vi "VMS_CameraRotator_Responder.vi"() -> ()   [LabVIEW 2018]
uses:
  <vilib>/rvi/Emulation/niFpgaGetClockAttributes.vi
  <vilib>/rvi/Emulation/niFpgaSctlEmulationGetInTimedLoop.vi
  <vilib>/rvi/Emulation/niFpgaEmulationReportErrorSimple.vi
  <vilib>/rvi/eio/common/nirviEmuTemplateMethod_errors.vi
  <vilib>/rvi/interface/RandomDataEmulation/niFpgaRandomDataHandleErrors.vi
  <vilib>/rvi/Emulation/niFpgaProcessEmulError.vi
  <vilib>/rvi/Emulation/niFpgaCriticalErrorInLSC.vi
  <vilib>/rvi/occurrence/nirviWaitOnOccurrenceBase.vi
  <vilib>/eio/EIOMethodNode/EIOMethodNode.xnode
  <vilib>/rvi/DataTransferAndStorage/Container/XNode/niFpgaContainer.xnode
  <vilib>/rvi/interface/RandomDataEmulation/nirviRandomDataFpgaReadWriteTemplate.vi
  <vilib>/eio/EIONode/EIONode.xnode
panel:
  out "Chassis Temperature":fxp<+/-,32,16>
  out "FIFO full":bool
  in  "Output type":i16
  in  "Period (ms)":u32=5
  out "Ready":bool
  out "Ticks":u64
  out "Timeouted":bool
  out "Stopped":bool
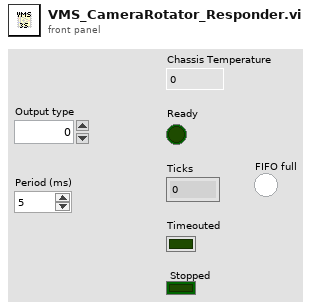
[diagram p1: front panel]
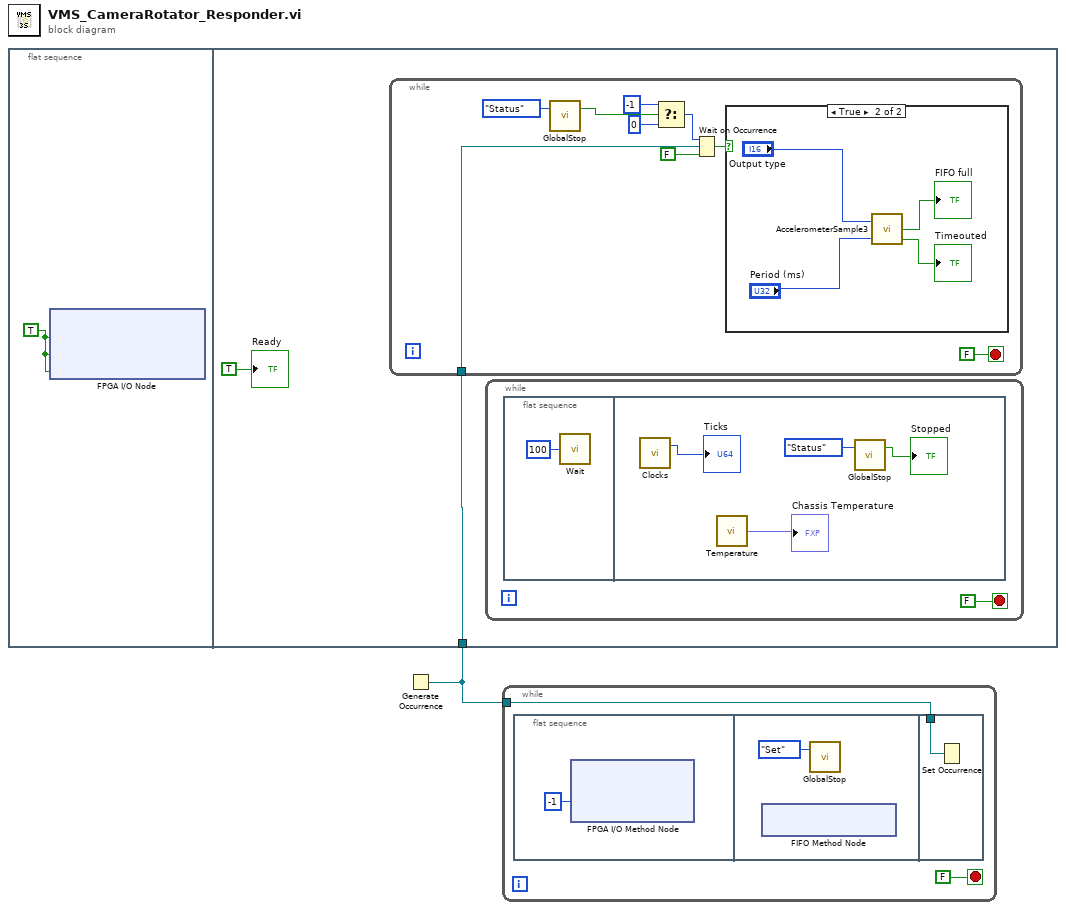
[diagram p0: block diagram]
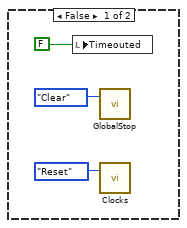
[diagram p2: hidden frame]
diagram:
  n1 = flat-sequence {
    tunnel: w1 -> [w3]
    frame #0 {
      w2 = TRUE ("Accelerometer5/Start")
      n2 = xnode "FPGA I/O Node"("Accelerometer1/Start"=w2, "Accelerometer2/Start"=w2, "Accelerometer3/Start"=w2) -> ()  [unwired: 3 in, 3 out]
    }
    frame #1 {
      n3 = while {
        tunnel: w3 -> [w17]
        stop <- FALSE stop-if-true
        n4 = call "GlobalStop.vi"("Enum"=enum16{"Clear", "Set", "Status"}."Status") -> ("Boolean"=w11:bool)  [unwired: 1 in, 1 out]
        n5 = Select(t=-1, s=w11, f=0) -> (s? t:f=w15:i32)
        n6 = Wait on Occurrence(1:FALSE ("ignore previous (T)"), 2:w17, 3:w15) -> (0:w18:bool)
        n7 = case shown="True" w18 {
          frame False {
            n8 = local write "Timeouted"(FALSE ("Timeouted")) -> ()
            n9 = call "GlobalStop.vi"("Enum"=enum16{"Clear", "Set", "Status"}."Clear") -> ()  [unwired: 1 in, 2 out]
            n10 = call "Clocks.vi"("Enum"=enum16{"Reset", "Increment", "Get"}."Reset") -> ()  [unwired: 1 in, 2 out]
          }
          frame True {
            n11 = call "AccelerometerSample3.vi"("Output type"="Output type", "Period (ms)"="Period (ms)") -> ("FIFO full"=→"FIFO full":bool, "Timeouted"=→"Timeouted":bool)  [unwired: 1 out]
          }
        }
      }
      n12 = while {
        stop <- FALSE stop-if-true
        n13 = flat-sequence {
          frame #0 {
            n14 = call "Wait"("Count(mSec)"=u32 100) -> ()  [unwired: 1 out]
          }
          frame #1 {
            n15 = call "Clocks.vi"() -> ("Clock"=→"Ticks":u64)  [unwired: 2 in, 1 out]
            n16 = call "Temperature.vi"() -> ("Mean temperature"=→"Chassis Temperature":fxp<+/-,32,16>)  [unwired: 1 in]
            n17 = call "GlobalStop.vi"("Enum"=enum16{"Clear", "Set", "Status"}."Status") -> ("Boolean"=→"Stopped":bool)  [unwired: 1 in, 1 out]
          }
        }
      }
      "Ready" <- TRUE ("Ready")
    }
  }
  n18 = Generate Occurrence() -> (w1:refnum<k4>)
  n19 = while {
    tunnel: w1 -> [w27]
    stop <- FALSE stop-if-true
    n20 = flat-sequence {
      tunnel: w27 -> [w31]
      frame #0 {
        n21 = xnode "FPGA I/O Method Node"("Timeout"=-1) -> ()  [unwired: 1 in, 2 out]
      }
      frame #1 {
        n22 = xnode ("FIFO Method Node")() -> ()  [unwired: 1 in, 1 out]
        n23 = call "GlobalStop.vi"("Enum"=enum16{"Clear", "Set", "Status"}."Set") -> ()  [unwired: 1 in, 2 out]
      }
      frame #2 {
        n24 = Set Occurrence(w31) -> ()
      }
    }
  }
